vi "Read Value.vi"(8 "error in (no error)":errorcluster, 11 "Optimiser Cell in":refnum<class "Optimiser Cell.lvclass">) -> (0 "error out":errorcluster, 2 "Value":dbl, 3 "Optimiser Cell out":refnum<class "Optimiser Cell.lvclass">)   [LabVIEW 2020, in "CIRCUS_uServices.lvlib" / "Run Utilities.lvlib" / "Optimiser Cell.lvclass"]
uses:
  Optimiser Cell.lvclass
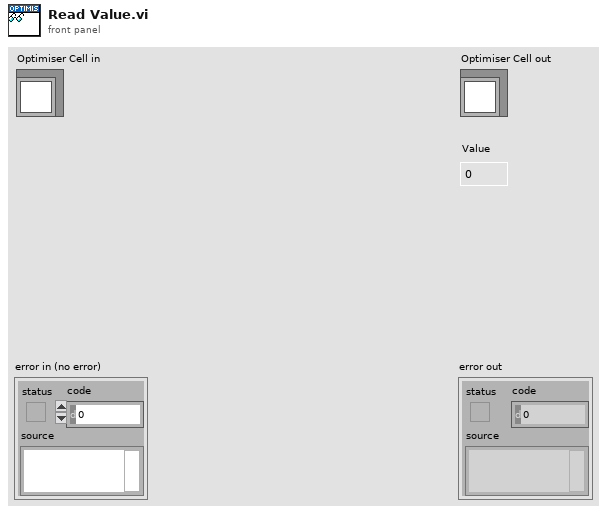
[diagram p1: front panel]
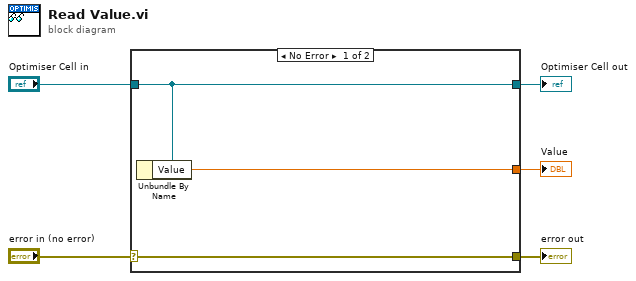
[diagram p0: block diagram]
diagram:
  n1 = case shown="No Error" "error in (no error)" {
    selector: "error in (no error)" -> [w8 w9]
    tunnel: [w8 w9] -> w4
    tunnel: [w7 w10] -> w2
    tunnel: "Optimiser Cell in" -> [w7 w10]
    tunnel: [w6 _] -> w1
    frame No Error {
      n2 = Unbundle By Name(w7) -> ("Value"=w6:dbl)
    }
    frame Error {
    }
  }
  "error out" <- w4
  "Optimiser Cell out" <- w2
  "Value" <- w1
